vi "Get Delimiter.vi"(8 "error in (no error)":errorcluster, 11 "Text Log File Specification in":refnum<class "Text Log File Specification.lvclass">) -> (0 "error out":errorcluster, 2 "Delimiter":string="\t", 3 "Text Log File Specification out":refnum<class "Text Log File Specification.lvclass">)   [LabVIEW 2015, in "Text Log File Specification.lvclass"]
uses:
  Text Log File Specification.lvclass
  Text Log File Specification.lvclass/Text Log File Specification.ctl
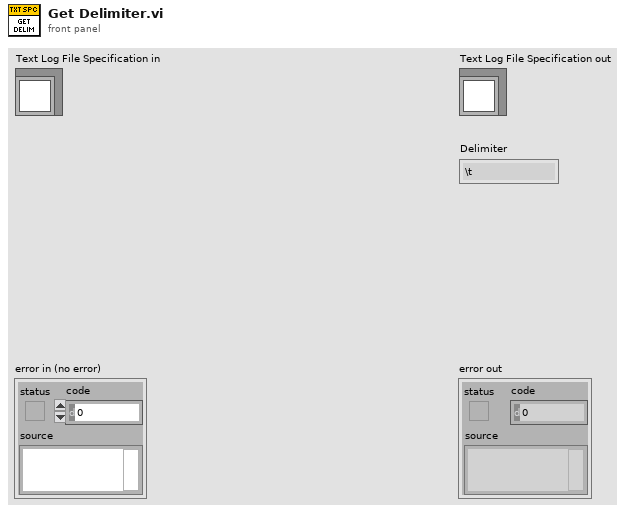
[diagram p1: front panel]
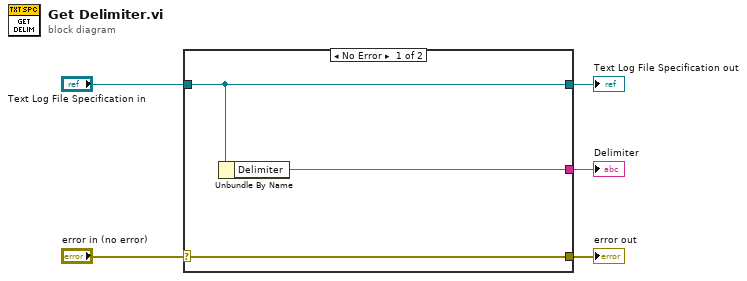
[diagram p0: block diagram]
diagram:
  n1 = case shown="No Error" "error in (no error)" {
    selector: "error in (no error)" -> [w8 w9]
    tunnel: [w8 w9] -> w4
    tunnel: [w7 w10] -> w2
    tunnel: "Text Log File Specification in" -> [w7 w10]
    tunnel: [w6 _] -> w1
    frame No Error {
      n2 = Unbundle By Name(w7) -> ("Delimiter"=w6:string)
    }
    frame Error {
    }
  }
  "error out" <- w4
  "Text Log File Specification out" <- w2
  "Delimiter" <- w1
